vi "Auto Griddy Score.vi"(8 "Command Info In":T1, 11 "Griddy Command":T4) -> (0 "Command Info Out":T1)   [LabVIEW 2020]
uses:
  Implementation/Typedefs/Teleop Manipulator Commands.ctl
  <vilib>/Rock Robotics/WPI/Framework/Command Status Info.ctl
  <vilib>/Rock Robotics/WPI/Framework/Completion Status.ctl
  <vilib>/Rock Robotics/WPI/Framework/Completion Notifier.ctl
  intake sub/Implementation/Typedef/intake typedef.ctl
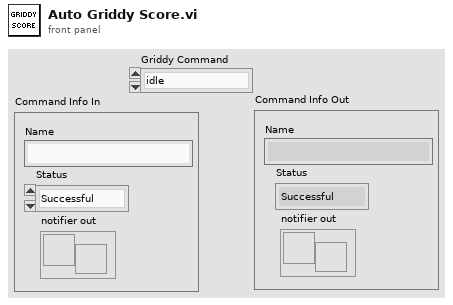
[diagram p1: front panel]
types:
  T1 = typedef "Command Status Info.ctl" = cluster{"Name":string, "Status":T2, "notifier out":T3}
  T2 = typedef "Completion Status.ctl" = enum16{"Successful", "Aborted", "Incomplete"}
  T3 = typedef "Completion Notifier.ctl" = refnum<notifier>
  T4 = typedef "Teleop Manipulator Commands.ctl" = enum16{"idle", "intake cone sideways", "intake cone upright", "intake cone feeder", "intake cube feeder", "intake cube", "score low cone", "score low cube", "score mid cone", "score mid cube", "score high cone", "score high cube", "score mid cone up"}
  T5 = typedef "intake typedef.ctl" = enum16{"Intake Cone Sideways", "Intake Cone Upright", "Intake Cube", "Outtake/Score", "Shoot"}
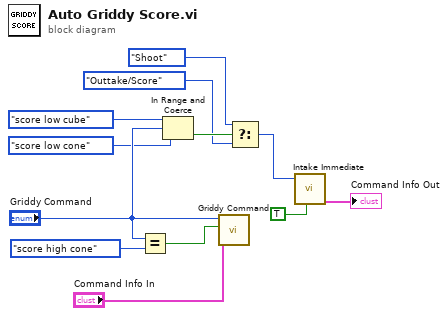
[diagram p0: block diagram]
diagram:
  n1 = Equal?(x="Griddy Command", y=Teleop_Manipulator_Commands."score high cone") -> (x = y?=w8:bool)
  n2 = In Range and Coerce(upper limit=Teleop_Manipulator_Commands."score low cube", x="Griddy Command", lower limit=Teleop_Manipulator_Commands."score low cone") -> (In Range?=w4:bool)  [unwired: 1 out]
  n3 = call "Griddy Command.vi"("Command Info In"="Command Info In", "Flip Wrist"=w8, "Griddy Command"="Griddy Command") -> ()  [unwired: 8 in, 1 out]
  n4 = Select(t=intake_typedef."Shoot" ("intake modes"), s=w4, f=intake_typedef."Outtake/Score" ("intake modes")) -> (s? t:f=w1:T5)
  n5 = call "Intake Immediate.vi"("Wait for Manipulator"=TRUE, "intake modes"=w1) -> ("Command Info Out"=→"Command Info Out":T1)  [unwired: 9 in]
